vi "percentInBand.vi"(9 "BandHalfWidth":dbl, 10 "targetPoints":dbl[](array[numeric]), 11 "matchPoints":dbl[](array[numeric])) -> (2 "percentInBand":dbl, 3 "inBand":i16[](array[numeric]))   [LabVIEW 2018]
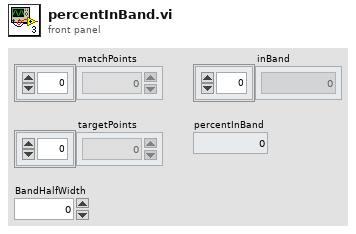
[diagram p1: front panel]
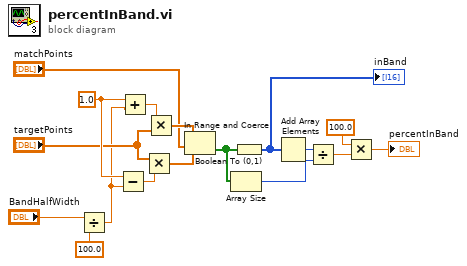
[diagram p0: block diagram]
diagram:
  w10 = 1.0
  n1 = Divide(x="BandHalfWidth", y=100.0) -> (x/y=w3:dbl)
  n2 = Subtract(x=w10, y=w3) -> (x-y=w8:dbl)
  n3 = Add(x=w10, y=w3) -> (x+y=w9:dbl)
  n4 = Multiply(x="targetPoints", y=w8) -> (x*y=w7:dbl[])
  n5 = Multiply(x=w9, y="targetPoints") -> (x*y=w6:dbl[])
  n6 = In Range and Coerce(upper limit=w6, x="matchPoints", lower limit=w7) -> (In Range?=w12:bool[])  [unwired: 1 out]
  n7 = Array Size(array=w12) -> (size(s)=w13:i32)
  n8 = Boolean To (0,1)(Boolean=w12) -> (0, 1=w17:i16[])
  "inBand" <- w17
  n9 = Add Array Elements(numeric array=w17) -> (sum=w11:i16)
  n10 = Divide(x=w11, y=w13) -> (x/y=w14:dbl)
  n11 = Multiply(x=100.0, y=w14) -> (x*y=→"percentInBand":dbl)
